vi "Write Single Coil Response.vi"(8 "error in (no error)":errorcluster, 10 "Modbus data unit in":refnum<class "Modbus Data Unit (PDU).lvclass">) -> (0 "error out":errorcluster, 1 "coil value":bool, 2 "address":u16)   [LabVIEW 2017, in "SubVIs.lvlib" / "Master Function Definition.lvlib"]
doc: "Decodes the response for the write single coil function."
uses:
  <vilib>/Modbus/subvis/Data and Functions/Master Function Definition/Master Function Definition.lvlib
  <vilib>/Modbus/subvis/Modbus Data Unit (PDU)/Modbus Data Unit (PDU).lvclass
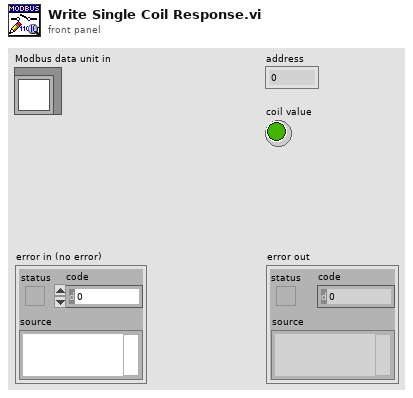
[diagram p1: front panel]
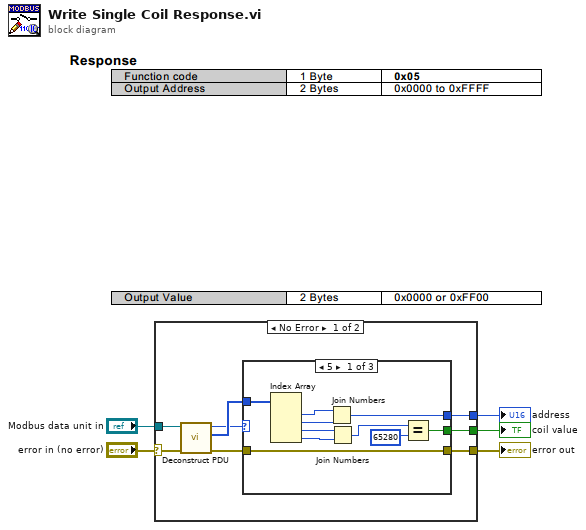
[diagram p0: block diagram]
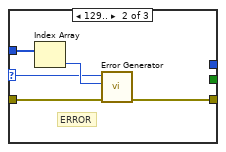
[diagram p2: hidden frame]
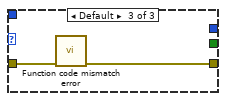
[diagram p3: hidden frame]
diagram:
  n1 = case shown="No Error" "error in (no error)" {
    selector: "error in (no error)" -> [w12 w31]
    tunnel: [w13 w31] -> w4
    tunnel: "Modbus data unit in" -> [w10 _]
    tunnel: [w8 _] -> w2
    tunnel: [w7 _] -> w1
    frame No Error {
      n2 = call <vilib>:"Deconstruct PDU.vi"("error in (no error)"=w12, "Modbus data unit in"=w10) -> ("error out"=w9:errorcluster, "data"=w11:u8[], "function"=w6:u8)  [unwired: 7 in]
      n3 = case shown="5" w6 {
        selector: w6 -> [_ w24 _]
        tunnel: w9 -> [w22 w25 w30]
        tunnel: w11 -> [w23 w28 _]
        tunnel: [w22 w27 w29] -> w13
        tunnel: [w21 _ _] -> w8
        tunnel: [w20 _ _] -> w7
        frame 5 {
          n4 = Index Array(array=w23) -> (element #1=w15:u8, element #2=w14:u8, element #3=w19:u8, element #4=w18:u8)  [unwired: 4 in]
          n5 = Join Numbers(hi=w15, lo=w14) -> ((hi.lo)=w20:u16)
          n6 = Join Numbers(hi=w19, lo=w18) -> ((hi.lo)=w16:u16)
          n7 = Equal?(x=w16, y=u16 65280) -> (x = y?=w21:bool)
        }
        frame 129.. {
          # "ERROR"
          n8 = Index Array(array=w28) -> (element=w26:u8)  [unwired: 1 in]
          n9 = call <vilib>:"Error Generator.vi"("error in (no error)"=w25, "data return (error code)"=w26, "function return"=w24) -> ("error out"=w27:errorcluster)  [unwired: 8 in]
        }
        frame Default {
          n10 = call <vilib>:"Function code mismatch error.vi"("error in (no error)"=w30) -> ("error out"=w29:errorcluster)  [unwired: 10 in]
        }
      }
    }
    frame Error {
    }
  }
  "error out" <- w4
  "coil value" <- w2
  "address" <- w1
